vi "LakeShore340 Control Panel.vi"(8 "error in (no error)":errorcluster, 11 "Class":refnum<class "LakeShore 340.lvclass">) -> (0 "error out":errorcluster, 3 "LakeShore 340 out":refnum<class "LakeShore 340.lvclass">)   [LabVIEW 2015, in "LakeShore 340.lvclass"]
uses:
  LakeShore 340.lvclass
  LakeShore340 Front Panel Data.ctl
  LakeShore340 Heater Ranges.ctl
  Neocera/Neocera Set Point Aproach.ctl
panel:
  in  "Data":T1={"Record heater"=FALSE, "A"=TRUE, "B"=FALSE, "Record RAW"=FALSE, "Set point"=0.0, "Set Heater Range"=enum."0 (Off)", "Approach"=enum."Instant", "Ramp rate, K/min"=0.0, "C"=FALSE, "D"=FALSE}
  # "Temperature Monitor"
  # "Record Channels"
  # "Temperature Control"
  # "1 A/50 Ohm\nsee manual\nfor rest"
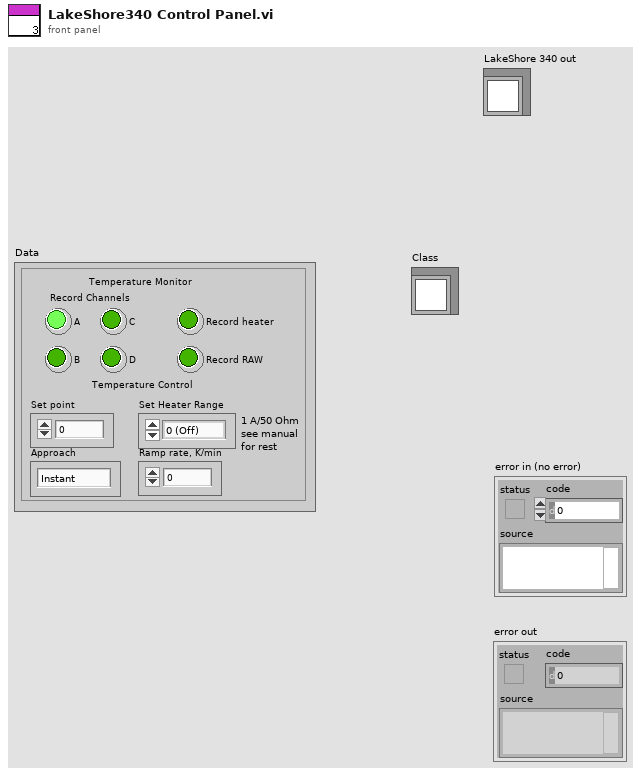
[diagram p1: front panel]
types:
  T1 = typedef "LakeShore340 Front Panel Data.ctl" = cluster{"Record heater":bool, "A":bool, "B":bool, "Record RAW":bool, "Set point":dbl, "Set Heater Range":T2, "Approach":T3, "Ramp rate, K/min":dbl, "C":bool, "D":bool}
  T2 = typedef "LakeShore340 Heater Ranges.ctl" = enum16{"0 (Off)", "1 (5 mW)", "2 (50 mW)", "3 (500 mW)", "4 (5 W)", "5 (50 W)"}
  T3 = typedef "Neocera Set Point Aproach.ctl" = enum16{"Instant", "Ramp"}
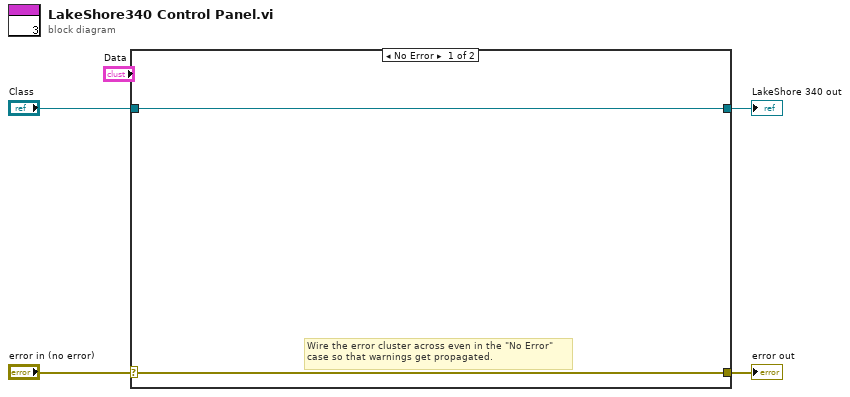
[diagram p0: block diagram]
diagram:
  n1 = case shown="No Error" "error in (no error)" {
    selector: "error in (no error)" -> [w5 w8]
    tunnel: [w5 w8] -> w3
    tunnel: [w6 w7] -> w1
    tunnel: "Class" -> [w6 w7]
    frame No Error {
      # "Wire the error cluster across even in the \"No Error\"\ncase so that warnings get propagated."
    }
    frame Error {
    }
  }
  "error out" <- w3
  "LakeShore 340 out" <- w1
